vi "Modbus Display Timer.vi"(5 "FVIR?":bool, 6 "Blower ON/OFF":bool, 7 "Counter of oil injections 1.1 cc/min":u16, 9 "Timing in":T2 {"Absolute Time" format="%<%H:%M:%S%3u>t"; "Display Time" format="%#.20f"; "Test Time Ref" format="%#.20f"; "Precondition Time Ref" format="%#.20f"; "First Call Time Ref" format="%#.20f"}, 10 "Absolute Time":dbl format="%#.20f", 11 "Real-Time Clock":T1) -> (1 "Timing Out":T2 {"Absolute Time" format="%<%H:%M:%S%3u>t"; "Display Time" format="%#.20f"; "Test Time Ref" format="%#.20f"; "Precondition Time Ref" format="%#.20f"; "First Call Time Ref" format="%#.20f"})   [LabVIEW 2020, in "Modbus.lvlib"]
uses:
  Modbus.lvlib
  Modbus Timing.ctl
  <vilib>/Utility/miscctls.llb/LVDateTimeRec.ctl
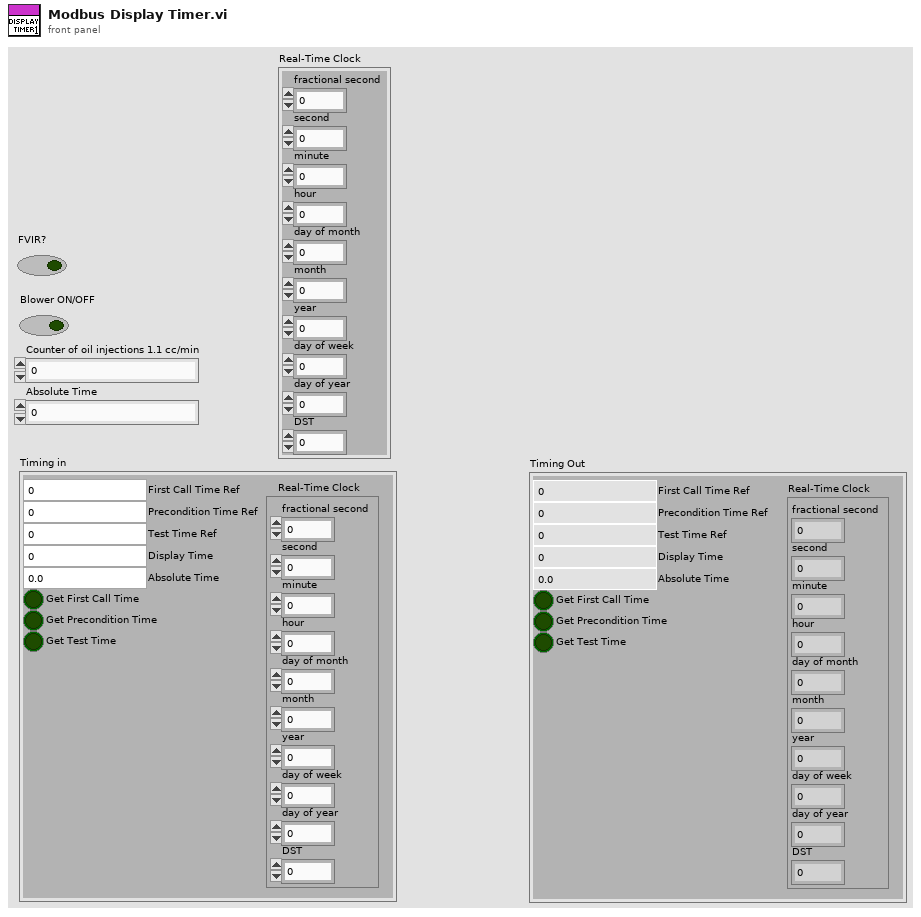
[diagram p1: front panel]
types:
  T1 = typedef "LVDateTimeRec.ctl" = cluster{"fractional second":dbl, "second":i32, "minute":i32, "hour":i32, "day of month":i32, "month":i32, "year":i32, "day of week":i32, "day of year":i32, "DST":i32}
  T2 = typedef "Modbus Timing.ctl" = cluster{"First Call Time Ref":dbl, "Precondition Time Ref":dbl, "Test Time Ref":dbl, "Get First Call Time":bool, "Get Precondition Time":bool, "Get Test Time":bool, "Display Time":dbl, "Real-Time Clock":T1, "Absolute Time":dbl}
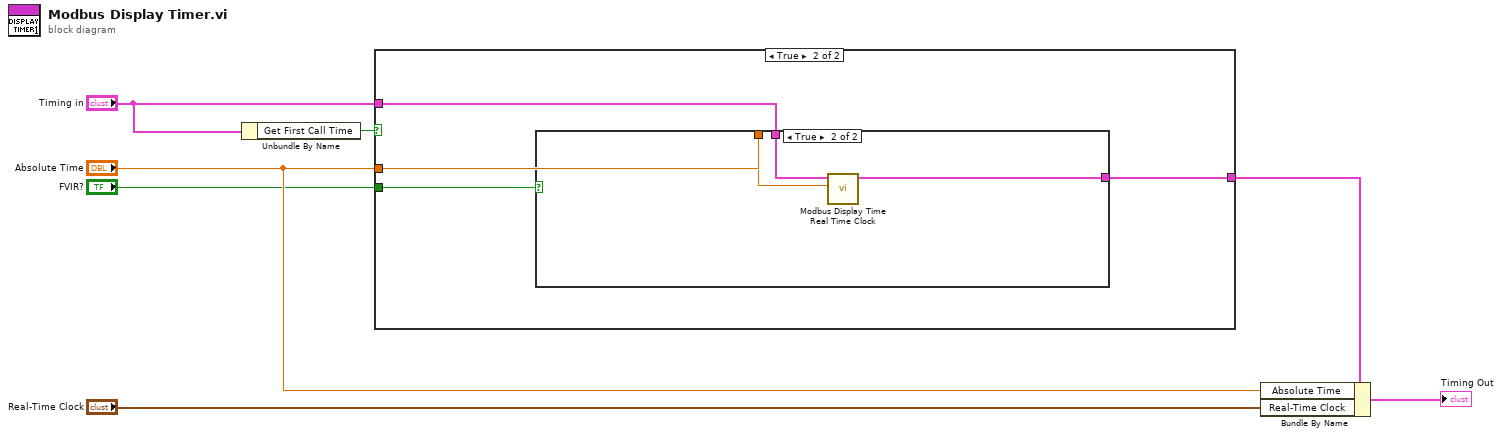
[diagram p0: block diagram]
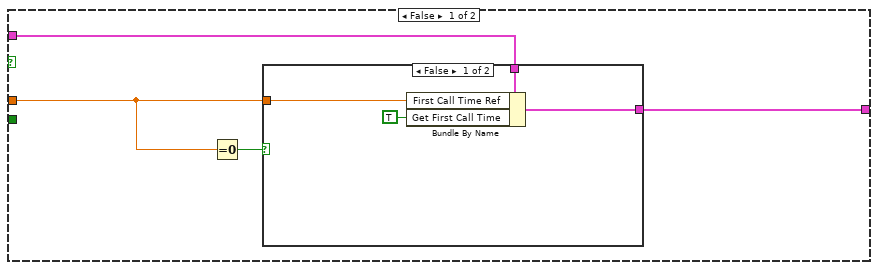
[diagram p2: hidden frame]
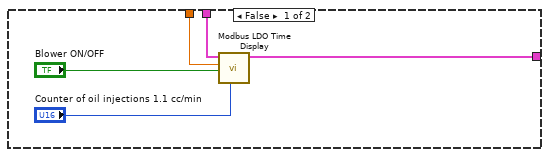
[diagram p4: hidden frame]
diagram:
  n1 = Unbundle By Name("Timing in") -> ("Get First Call Time"=w6:bool)
  n2 = case shown="True" w6 {
    tunnel: "Timing in" -> [w11 w19]
    tunnel: "Absolute Time" -> [w9 w20]
    tunnel: [w10 w18] -> w5
    tunnel: "FVIR?" -> [_ w17]
    frame False {
      n3 = Equal To 0?(x=w9) -> (x = 0?=w8:bool)
      n4 = case shown="False" w8 {
        tunnel: w11 -> [w15 w16]
        tunnel: [w14 w16] -> w10
        tunnel: w9 -> [w12 _]
        frame False {
          n5 = Bundle By Name(cluster=w15, "First Call Time Ref"=w12, "Get First Call Time"=TRUE) -> (w14:T2)
        }
        frame True {
        }
      }
    }
    frame True {
      n6 = case shown="True" w17 {
        tunnel: w20 -> [w25 w26]
        tunnel: w19 -> [w24 w28]
        tunnel: [w23 w27] -> w18
        frame False {
          n7 = call "Modbus LDO Time Display.vi"("Counter of oil injections 1.1 cc/min"="Counter of oil injections 1.1 cc/min", "Blower ON/OFF"="Blower ON/OFF", "Absolute Time"=w25, "Timing in"=w24) -> ("Timing Out"=w23:T2)  [unwired: 7 in]
        }
        frame True {
          n8 = call "Modbus Display Time Real Time Clock.vi"("Absolute Time"=w26, "Timing in in"=w28) -> ("Timing out"=w27:T2)  [unwired: 9 in]
        }
      }
    }
  }
  n9 = Bundle By Name(cluster=w5, "Absolute Time"="Absolute Time", "Real-Time Clock"="Real-Time Clock") -> (→"Timing Out":T2)
